vi "Instrumento virtual.vi"() -> ()   [LabVIEW 2020]
uses:
  <vilib>/Instr/_visa.llb/VISA Configure Serial Port (Instr).vi
  <vilib>/Utility/file.llb/Write Delimited Spreadsheet (DBL).vi
panel:
  out "Numeric":dbl
  out "CB":cluster{"R raw":i32, "G raw":i32, "B raw":i32}
  out "CW":cluster{"R raw":i32, "G raw":i32, "B raw":i32}
  in  "CSV file":path
  out "R":dbl
  out "B":dbl
  out "G":dbl
  in  "Save sample":bool
  out "current time":timestamp
  in  "?":u16(slide) scale=0.0..250.0
  out "Waveform Graph":waveform(dbl)[](graph)
  out "Last saved sample":u32(colorbox)
  in  "White\nWhite":bool
  in  "Black":bool
  out "B raw":i32
  out "G raw":i32
  out "R raw":i32
  in  "Serial Port":refnum<visa-resource-name>
  out "Current Box":u32(colorbox)
  in  "?":bool
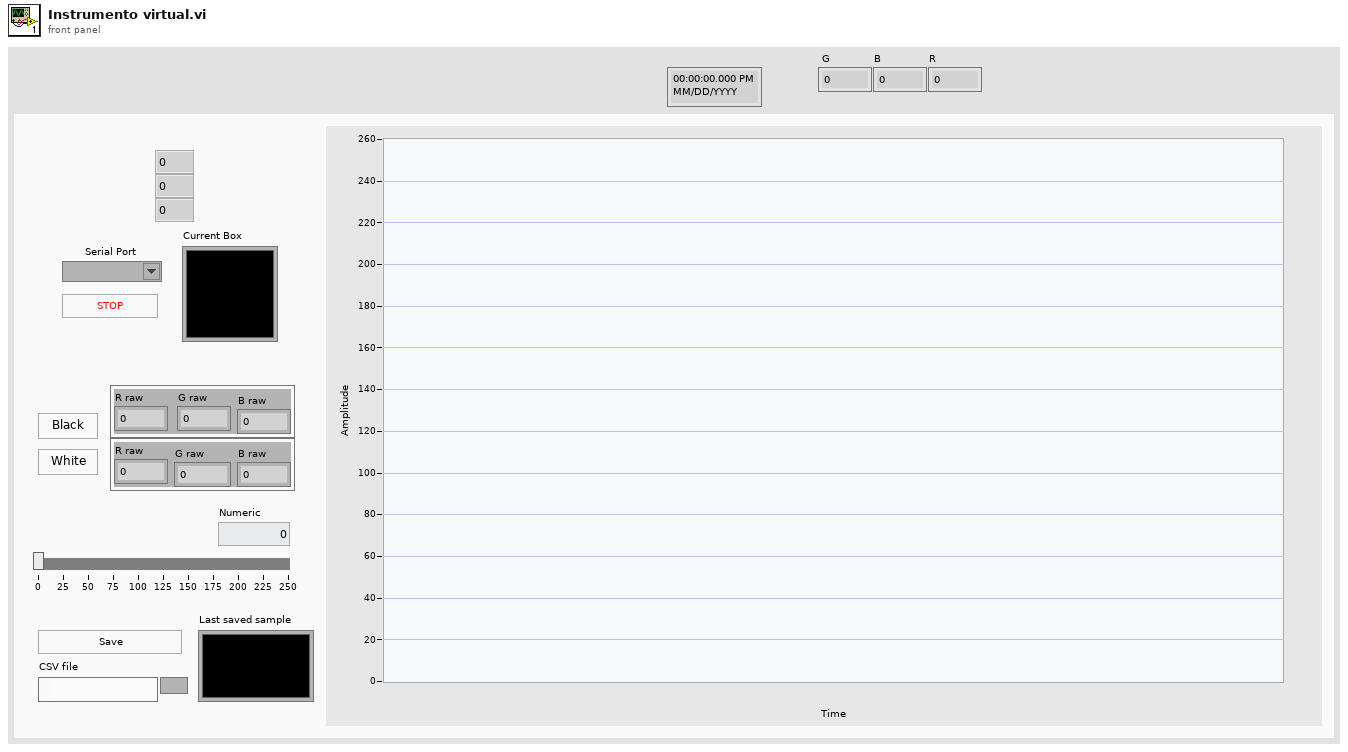
[diagram p1: front panel]
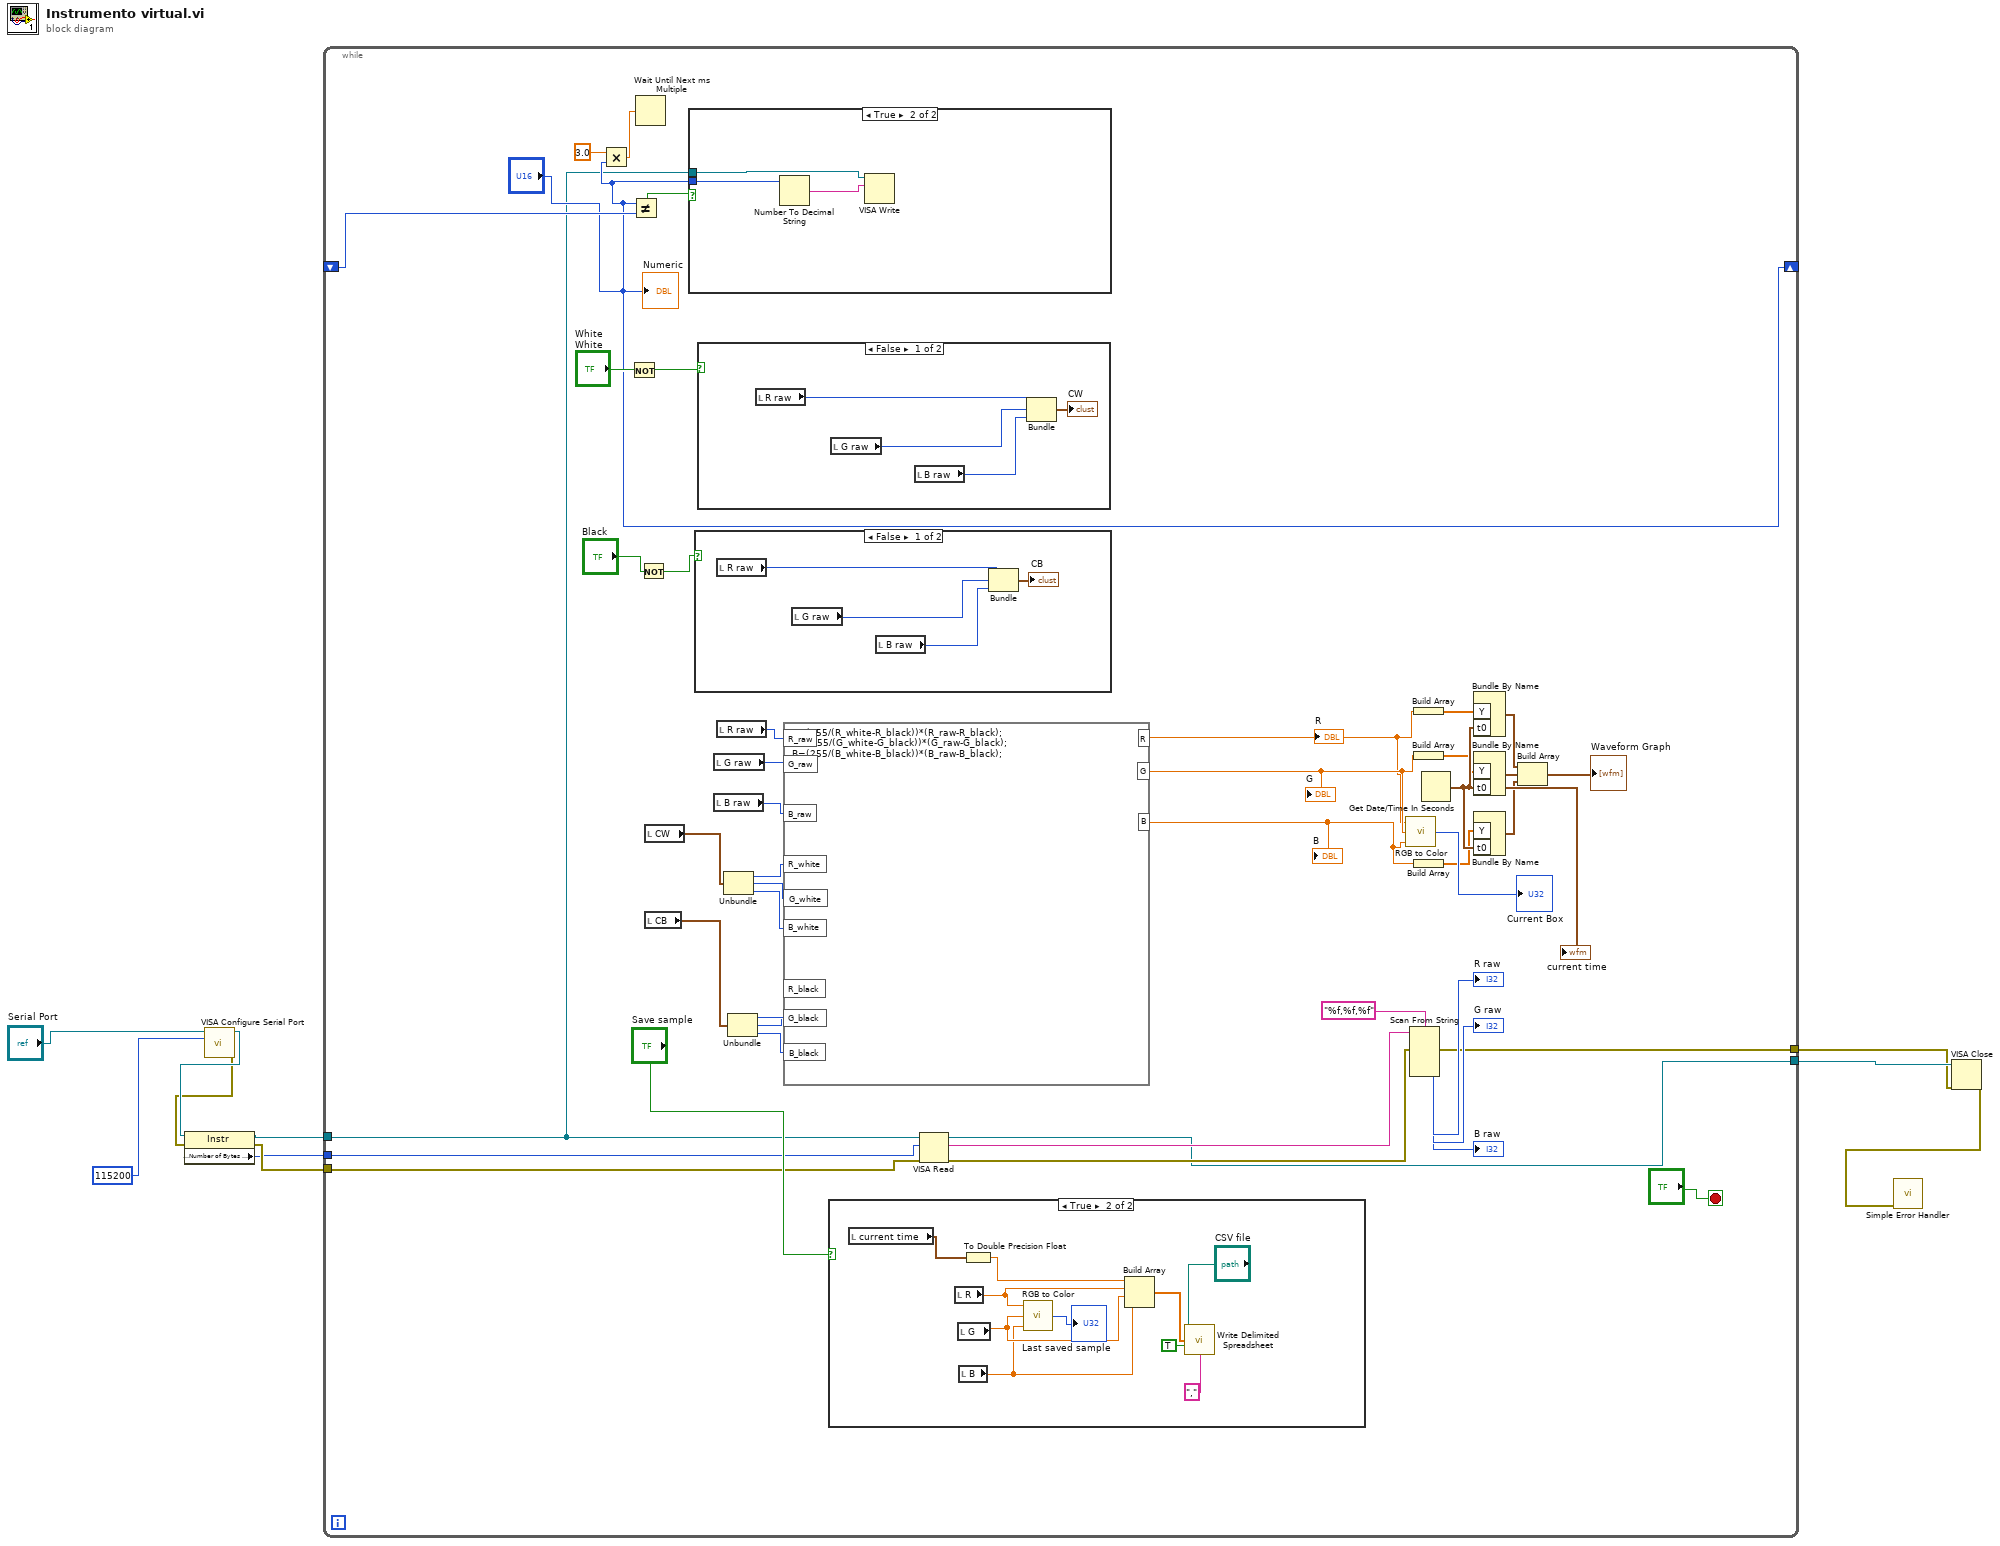
[diagram p0: block diagram]
diagram:
  n1 = call-poly "VISA Configure Serial Port"("VISA resource name"="Serial Port", "baud rate (9600)"=u32 115200) -> ("VISA resource name out"=w4:refnum<visa-resource-name>, "error out"=w3:errorcluster)  [unwired: 12 in]
  n2 = property class="Instr"(reference=w4, error in=w3) -> (reference out=w6:refnum<visa-resource-name>, error out=w5:errorcluster, "Serial Settings:Number of Bytes at Serial Port"=w2:u32)
  n3 = while {
    shift-right: ["?"] -> _
    shift-left: _ -> [w14]
    tunnel: [w17] -> w8
    tunnel: [w16] -> w7
    tunnel: w6 -> [w11]
    tunnel: w5 -> [w15]
    tunnel: w2 -> [w13]
    stop <- "?" stop-if-true
    n4 = Multiply(x=3.0, y="?") -> (x*y=w18:dbl)
    n5 = Not(x="White\nWhite") -> (.not. x?=w32:bool)
    n6 = Not Equal?(x="?", y=w14) -> (x != y?=w20:bool)
    n7 = Wait Until Next ms Multiple(millisecond multiple=w18) -> ()  [unwired: 1 out]
    n8 = Not(x="Black") -> (.not. x?=w29:bool)
    n9 = local read "CW"() -> (w28:cluster{"R raw":i32, "G raw":i32, "B raw":i32})
    n10 = local read "CB"() -> (w27:cluster{"R raw":i32, "G raw":i32, "B raw":i32})
    n11 = case shown="True" w20 {
      tunnel: "?" -> [_ w58]
      tunnel: w11 -> [_ w56]
      frame False {
      }
      frame True {
        n12 = Number To Decimal String(number=w58) -> (decimal integer string=w57:string)  [unwired: 1 in]
        n13 = VISA Write(VISA resource name=w56, write buffer=w57) -> ()  [unwired: 1 in, 3 out]
      }
    }
    n14 = case shown="False" w29 {
      frame False {
        n15 = local read "R raw"() -> (w73:i32)
        n16 = local read "G raw"() -> (w74:i32)
        n17 = local read "B raw"() -> (w75:i32)
        n18 = Bundle("R raw"=w73, "G raw"=w74, "B raw"=w75) -> (→"CB":cluster{"R raw":i32, "G raw":i32, "B raw":i32})  [unwired: 1 in]
      }
      frame True {
      }
    }
    n19 = case shown="False" w32 {
      frame False {
        n20 = local read "R raw"() -> (w72:i32)
        n21 = local read "G raw"() -> (w71:i32)
        n22 = local read "B raw"() -> (w70:i32)
        n23 = Bundle("R raw"=w72, "G raw"=w71, "B raw"=w70) -> (→"CW":cluster{"R raw":i32, "G raw":i32, "B raw":i32})  [unwired: 1 in]
      }
      frame True {
      }
    }
    n24 = local read "G raw"() -> (w41:i32)
    n25 = local read "B raw"() -> (w40:i32)
    n26 = local read "R raw"() -> (w42:i32)
    n27 = Unbundle(w28) -> ("R raw"=w26:i32, "G raw"=w25:i32, "B raw"=w24:i32)
    n28 = Unbundle(w27) -> ("R raw"=w23:i32, "G raw"=w22:i32, "B raw"=w21:i32)
    n29 = formula code="R=(255/(R_white-R_black))*(R_raw-R_black);\nG=(255/(G_white-G_black))*(G_raw-G_black);\nB=(255/(B_white-B_black))*(B_raw-B_black);"("R_raw"=w42, "G_raw"=w41, "B_raw"=w40, "R_white"=w26, "G_white"=w25, "B_white"=w24, "R_black"=w23, "G_black"=w22, "B_black"=w21) -> ("R"=w35:dbl, "G"=w36:dbl, "B"=w37:dbl)
    "G" <- w36
    "B" <- w37
    "R" <- w35
    n30 = case shown="True" "Save sample" {
      frame False {
      }
      frame True {
        n31 = local read "current time"() -> (w67:timestamp)
        n32 = local read "R"() -> (w66:dbl)
        n33 = local read "G"() -> (w65:dbl)
        n34 = local read "B"() -> (w64:dbl)
        n35 = To Double Precision Float(number=w67) -> (double precision float=w68:dbl)
        n36 = call <vilib>:"RGB to Color.vi"("B"=w64, "G"=w65, "R"=w66) -> ("Color"=→"Last saved sample":u32)
        n37 = Build Array(w68, w66, w65, w64) -> (w61:dbl[])
        n38 = call-poly <vilib>:"Write Delimited Spreadsheet.vi"("file path (dialog if empty)"="CSV file", "1D data"=w61, "append to file? (new file:F)"=TRUE, "delimiter (\\t)"="," ("delimiter (\\t)")) -> ()  [unwired: 10 in, 2 out]
      }
    }
    n39 = VISA Read(VISA resource name=w11, byte count=w13, error in (no error)=w15) -> (VISA resource name out=w17:refnum<visa-resource-name>, read buffer=w45:string, error out=w44:errorcluster)  [unwired: 1 out]
    n40 = call <vilib>:"RGB to Color.vi"("B"=w37, "G"=w36, "R"=w35) -> ("Color"=→"Current Box":u32)
    n41 = Scan From String(format string="%f,%f,%f", input string=w45, error in=w44) -> (error out=w16:errorcluster, output 1=→"R raw":i32, output 2=→"G raw":i32, output 3=→"B raw":i32)  [unwired: 4 in, 2 out]
    n42 = Build Array(w35) -> (w39:dbl[])
    n43 = Build Array(w36) -> (w38:dbl[])
    n44 = Build Array(w37) -> (w34:dbl[])
    n45 = Get Date/Time In Seconds() -> (seconds since 1Jan1904=w51:timestamp)
    "current time" <- w51
    n46 = Bundle By Name("Y"=w39, "t0"=w51) -> (w49:waveform(dbl))  [unwired: 1 in]
    n47 = Bundle By Name("Y"=w38, "t0"=w51) -> (w47:waveform(dbl))  [unwired: 1 in]
    n48 = Bundle By Name("Y"=w34, "t0"=w51) -> (w46:waveform(dbl))  [unwired: 1 in]
    n49 = Build Array(w49, w47, w46) -> (→"Waveform Graph":waveform(dbl)[])
    "Numeric" <- "?"
  }
  n50 = VISA Close(VISA resource name=w8, error in (no error)=w7) -> (error out=w10:errorcluster)
  n51 = call <vilib>:"Simple Error Handler.vi"("error in (no error)"=w10) -> ()  [unwired: 1 in, 8 out]
